vi "AI init.vi"(10 "N_param":i32) -> (0 "error":errorcluster, 3 "AI":T1)   [LabVIEW 2019, in "Inputs.lvlib"]
uses:
  Inputs.lvlib
  Ctl/AI.ctl
  Ctl/AI short.ctl
  Ctl/Parameter State.ctl
panel:
  # "Analog parameters"
  # "Description of analog parameters"
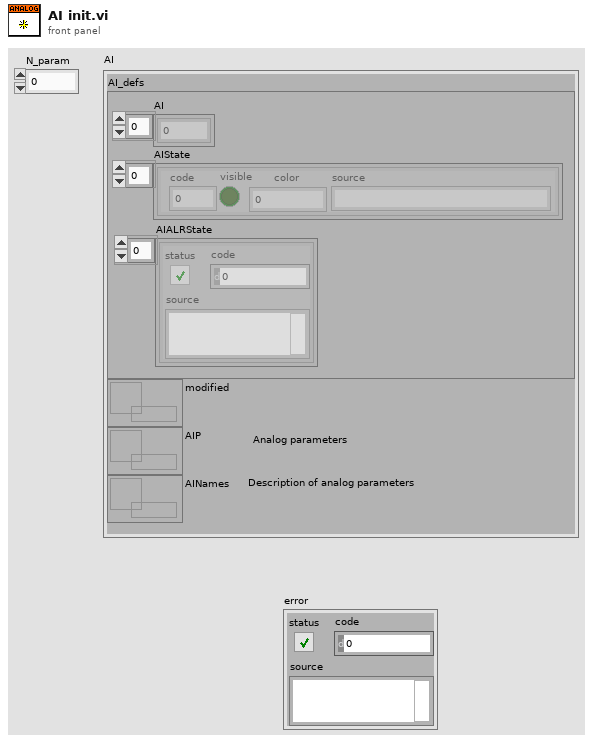
[diagram p1: front panel]
types:
  T1 = typedef "Inputs.lvlib/AI.ctl" = cluster{"AI_defs":T2, "modified":refnum<data-value>, "AIP":refnum<data-value>, "AINames":refnum<data-value>}
  T2 = typedef "Inputs.lvlib/AI short.ctl" = cluster{"AI":dbl[], "AIState":T3[], "AIALRState":errorcluster[]}
  T3 = typedef "Inputs.lvlib/Parameter State.ctl" = cluster{"code":i32, "visible":bool, "color":u32, "source":string}
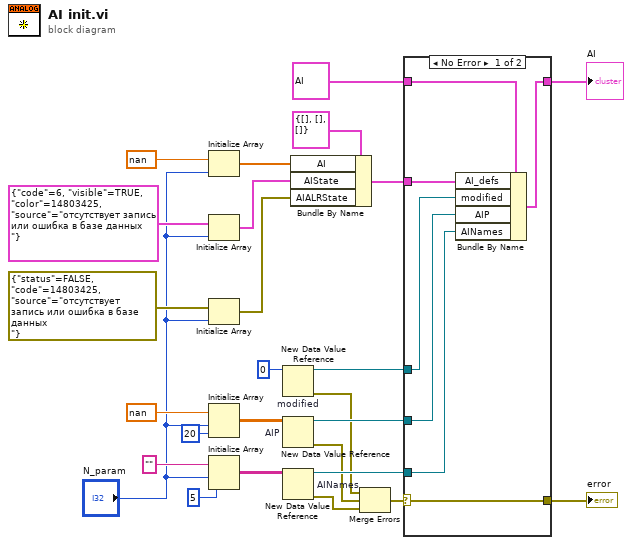
[diagram p0: block diagram]
diagram:
  n1 = Initialize Array(nan ("PV"), "N_param") -> (w24:dbl[])
  n2 = Initialize Array(T3 {"code"=6, "visible"=TRUE, "color"=14803425, "source"="отсутствует запись или ошибка в базе данных                                                                                    "} ("STATE"), "N_param") -> (w23:T3[])
  n3 = Initialize Array(errorcluster {"status"=FALSE, "code"=14803425, "source"="отсутствует запись или ошибка в базе данных                                                                                    "} ("ALRSTATE"), "N_param") -> (w22:errorcluster[])
  n4 = Initialize Array(nan ("AIP"), "N_param", 20 ("dimension size")) -> (w7:dbl[][])
  n5 = Initialize Array("" ("AINames"), "N_param", 5 ("dimension size")) -> (w16:string[][])
  n6 = New Data Value Reference "modified"(data value=u8 0 ("modified")) -> (data value reference=w2:refnum<data-value>, error out=w3:errorcluster)  [unwired: 1 in]
  n7 = New Data Value Reference "AIP"(data value=w7) -> (data value reference=w6:refnum<data-value>, error out=w4:errorcluster)  [unwired: 1 in]
  n8 = New Data Value Reference "AINames"(data value=w16) -> (data value reference=w15:refnum<data-value>, error out=w8:errorcluster)  [unwired: 1 in]
  n9 = Bundle By Name(cluster=T2 {"AI"=[], "AIState"=[], "AIALRState"=[]} ("AI_defs"), "AI"=w24, "AIState"=w23, "AIALRState"=w22) -> (w11:T2)
  n10 = Merge Errors(w3, w4, w8) -> (w5:errorcluster)
  n11 = case shown="No Error" w5 {
    selector: w5 -> [w30 w35]
    tunnel: w6 -> [w28 _]
    tunnel: w15 -> [w29 _]
    tunnel: [w30 w35] -> w13
    tunnel: w11 -> [w32 _]
    tunnel: T1 {"AI_defs"={"AI"=[], "AIState"=[], "AIALRState"=[]}, "modified"=refnum, "AIP"=refnum, "AINames"=refnum} ("AI") -> [w33 w34]
    tunnel: [w31 w34] -> w9
    tunnel: w2 -> [w27 _]
    frame No Error {
      n12 = Bundle By Name(cluster=w33, "AI_defs"=w32, "modified"=w27, "AIP"=w28, "AINames"=w29) -> (w31:T1)
    }
    frame Error {
    }
  }
  "error" <- w13
  "AI" <- w9
